vi "EMV T6 Indicating Flow.vi"(8 "error in (no error)":errorcluster, 10 "T6_DELTA_INDICATING_FLOW":dbl=2.0, 11 "Mixing Valve.T6 Temp (0x406E)":dbl) -> (0 "error out":errorcluster, 3 "Flow Dectection":bool)   [LabVIEW 2016]
panel:
  out "First - Row 10":dbl
  out "T6 History":dbl[](array[numeric])
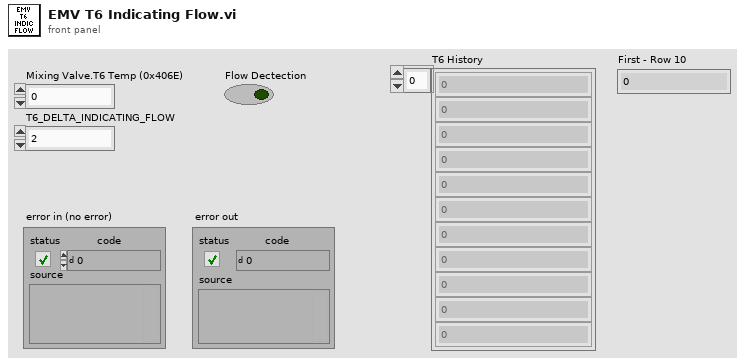
[diagram p1: front panel]
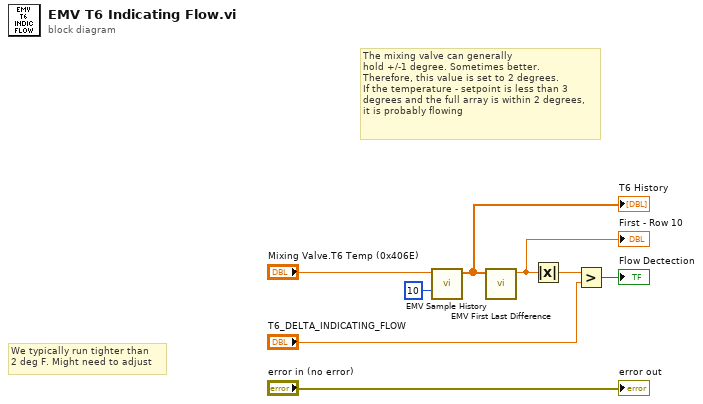
[diagram p0: block diagram]
diagram:
  # "We typically run tighter than \n2 deg F. Might need to adjust"
  # "The mixing valve can generally\nhold +/-1 degree. Sometimes better.\nTherefore, this value is set to 2 degrees. \nIf the temperature - setpoint is less than 3\ndegrees and the full array is within 2 degrees,\nit is probably flowing"
  n1 = call "EMV Sample History.vi"("length"=10, "T6 Temp"="Mixing Valve.T6 Temp (0x406E)") -> ("T6 History"=w3:dbl[])  [unwired: 8 in, 1 out]
  "T6 History" <- w3
  n2 = call "EMV First Last Difference.vi"("Current T6 Temperatures in"=w3) -> ("First - Row 10"=w7:dbl)  [unwired: 6 in, 4 out]
  "First - Row 10" <- w7
  n3 = Absolute Value(x=w7) -> (abs(x)=w8:dbl)
  n4 = Greater?(x=w8, y="T6_DELTA_INDICATING_FLOW") -> (0:→"Flow Dectection":bool)
  "error out" <- "error in (no error)"
